vi "pi.calculate_trapezoidal.vi"(6 "sampling_time (s)":dbl, 10 "Ti":dbl, 11 "Kc":dbl) -> (2 "a1...an":dbl[](array[numeric]), 3 "b0...bn":dbl[](array[numeric]))   [LabVIEW 2015, in "discrete_control_systems.lvlib"]
doc: "Calculates the gains for a discrete difference equation from the PI controller parameters using the trapezoidal discretization method.\n\nThe implemented controller has the following equation in the LaPlace domain, where U(s) is the controller output:\n\nU(s) = Kc * ( 1 + 1/(Ti*s) )"
uses:
  discrete_control_systems.lvlib
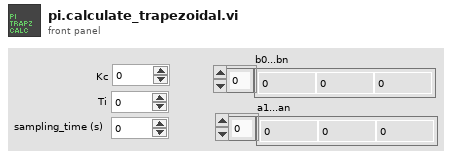
[diagram p1: front panel]
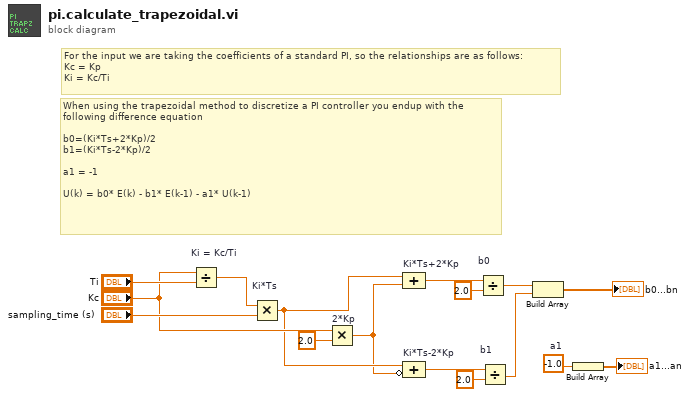
[diagram p0: block diagram]
diagram:
  w14 = -1.0  # a1
  # "For the input we are taking the coefficients of a standard PI, so the relationships are as follows:\nKc = Kp\nKi = Kc/Ti"
  # "When using the trapezoidal method to discretize a PI controller you endup with the\nfollowing difference equation\n\nb0=(Ki*Ts+2*Kp)/2\nb1=(Ki*Ts-2*Kp)/2\n\na1 = -1\n\nU(k) = b0* E(k) - b1* E(k-1) - a1* U(k-1)"
  n1 = Divide "Ki = Kc/Ti"(x="Kc", y="Ti") -> (x/y=w15:dbl)
  n2 = Multiply "Ki*Ts"(x=w15, y="sampling_time (s)") -> (x*y=w5:dbl)
  n3 = Multiply "2*Kp"(x="Kc", y=2.0) -> (x*y=w4:dbl)
  n4 = Compound Arithmetic op=ADD "Ki*Ts+2*Kp"(w5, w4) -> (w8:dbl)
  n5 = Compound Arithmetic op=ADD "Ki*Ts-2*Kp"(w5, invert w4) -> (w2:dbl)
  n6 = Divide "b0"(x=w8, y=2.0) -> (x/y=w6:dbl)
  n7 = Divide "b1"(x=w2, y=2.0) -> (x/y=w1:dbl)
  n8 = Build Array(w6, w1) -> (→"b0...bn":dbl[])
  n9 = Build Array(w14) -> (→"a1...an":dbl[])
